vi "Read Script Name.vi"(11 "Job Initialize in":refnum<class "Job Initialize.lvclass">) -> (2 "Script Name":string)   [LabVIEW 2014, in "Job Initialize.lvclass"]
uses:
  Job Initialize.lvclass
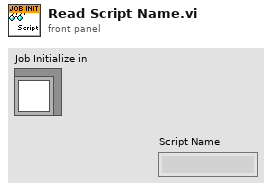
[diagram p1: front panel]
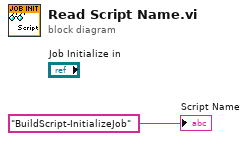
[diagram p0: block diagram]
diagram:
  "Script Name" <- "BuildScript-InitializeJob" ("Script Job Name")
